vi "getMagnetVector.vi"(8 "error in (no error)":errorcluster, 11 "Instrument.Cryostat in":refnum<class "Instrument.Cryostat.lvclass">) -> (0 "error out":errorcluster, 1 "Status":string, 2 "Field (T)":dbl[](array[numeric]), 3 "Instrument.Cryostat out":refnum<class "Instrument.Cryostat.lvclass">, 4 "Finished?":bool)   [LabVIEW 2019, in "Instrument.Cryostat.lvclass"]
uses:
  Instrument.Cryostat.lvclass
  C:/Users/patrick/Documents/GitHub/Instrument-Framework/lvsrc/Instrument/Instrument.lvclass
  Typedefs/getMagnetVector--cluster.ctl
  Typedefs/Cryostat.commands--enum.ctl
  de734779-1238-4c0a-9bbe-773738903950.vi
  de734779-1238-4c0a-9bbe-773738903950.vi/ddf619e1-382e-43de-b6b8-ddd34f231e73.vi
  de734779-1238-4c0a-9bbe-773738903950.vi/ddf619e1-382e-43de-b6b8-ddd34f231e73.vi/9757bebf-9d52-4042-8c77-42bd7329fc72.vi
  de734779-1238-4c0a-9bbe-773738903950.vi/ddf619e1-382e-43de-b6b8-ddd34f231e73.vi/88260920-64cd-45aa-bdf7-9047a73fd538.vi
  Instrument/Protected/Validate API method.vi
  Instrument/Private/Get RC Connection Status.vi
  Instrument/API/Send and Receive.vi
  <vilib>/Utility/Data Type/Get Type Information.vi
  <vilib>/JDP Science/JSONtext/JSON text to Variant.vi
  <vilib>/JDP Science/JSONtext/LVClass Serializer/JSONtext LVClass Serializer.lvclass
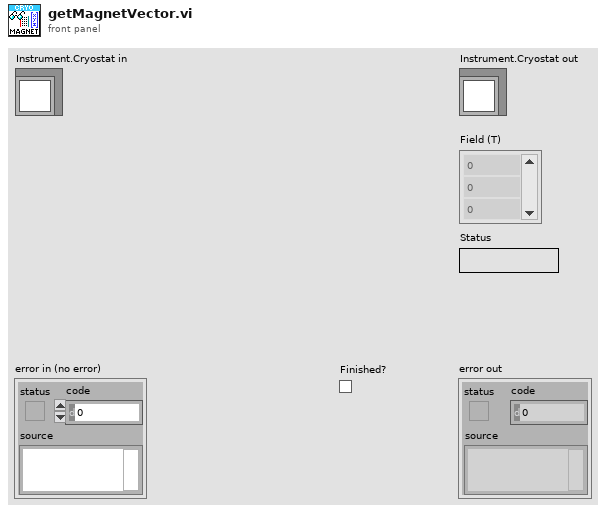
[diagram p1: front panel]
types:
  T1 = typedef "Instrument.Cryostat.lvclass/Cryostat.commands--enum.ctl" = enum16{"getLN2Level", "getLHeLevel", "getMagnet", "getMagnetVector", "setMagnet", "setMagnetVector", "getAngle", "setAngle", "getTemperature", "setTemperature", "getHeater", "setHeater", "getChamber", "setChamber", "getPressure"}
  T2 = typedef "Instrument.Cryostat.lvclass/getMagnetVector--cluster.ctl" = cluster{"field":dbl[], "status":string, "finished":bool}
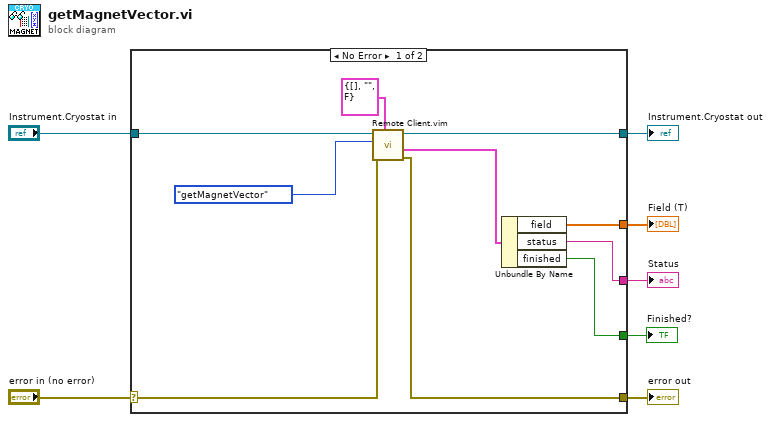
[diagram p0: block diagram]
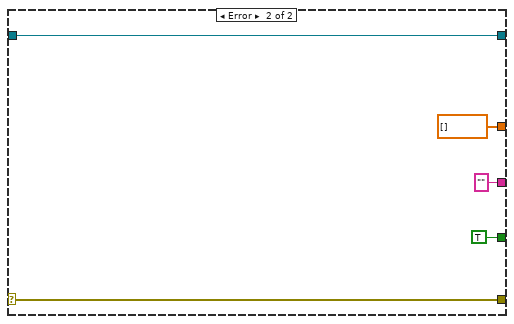
[diagram p2: hidden frame]
diagram:
  n1 = case shown="No Error" "error in (no error)" {
    selector: "error in (no error)" -> [w9 w22]
    tunnel: [w12 w22] -> w6
    tunnel: [w17 w21] -> w4
    tunnel: "Instrument.Cryostat in" -> [w10 w21]
    tunnel: [w16 dbl[] [] ("Field (T)")] -> w3
    tunnel: [w15 "" ("Status")] -> w2
    tunnel: [w14 TRUE] -> w1
    frame No Error {
      n2 = call "Remote Client.vim"("Data Out type"=T2 {"field"=[], "status"="", "finished"=FALSE} ("getMagnet"), "error in (no error)"=w9, "Command in"=Cryostat.commands--enum."getMagnetVector" ("commands"), "Instrument in"=w10) -> ("error out"=w12:errorcluster, "Data out"=w13:T2, "Instrument out"=w17:refnum<class "Instrument.Cryostat.lvclass">)  [unwired: 4 in, 1 out]
      n3 = Unbundle By Name(w13) -> ("field"=w16:dbl[], "status"=w15:string, "finished"=w14:bool)
    }
    frame Error {
    }
  }
  "error out" <- w6
  "Instrument.Cryostat out" <- w4
  "Field (T)" <- w3
  "Status" <- w2
  "Finished?" <- w1
